vi "Trama_GSA(SubVI).vi"(0 "TRAMA":string) -> (1 "Cluster":T2, 2 "3D fix":string, 3 "Cluster 2":T1)   [LabVIEW 2020]
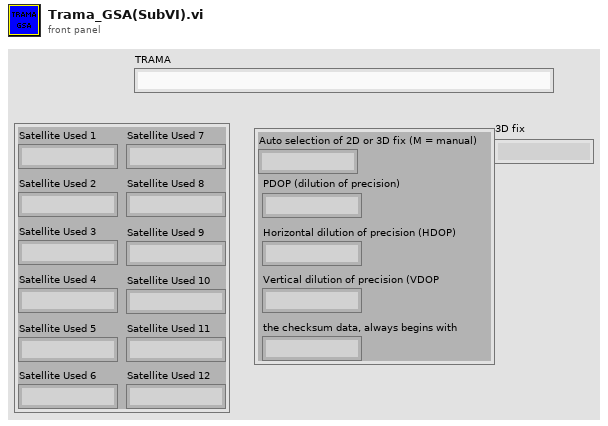
[diagram p1: front panel]
types:
  T1 = cluster{"Satellite Used 1":string, "Satellite Used 2":string, "Satellite Used 3":string, "Satellite Used 4":string, "Satellite Used 5":string, "Satellite Used 6":string, "Satellite Used 7":string, "Satellite Used 8":string, "Satellite Used 9":string, "Satellite Used 10":string, "Satellite Used 11":string, "Satellite Used 12":string}
  T2 = cluster{"Auto selection of 2D or 3D fix (M = manual)":string, "PDOP (dilution of precision)":string, "Horizontal dilution of precision (HDOP)":string, "Vertical dilution of precision (VDOP":string, "the checksum data, always begins with":string}
  T3 = cluster{string, string, string, string, string, string, string, string, string, string, string, string}
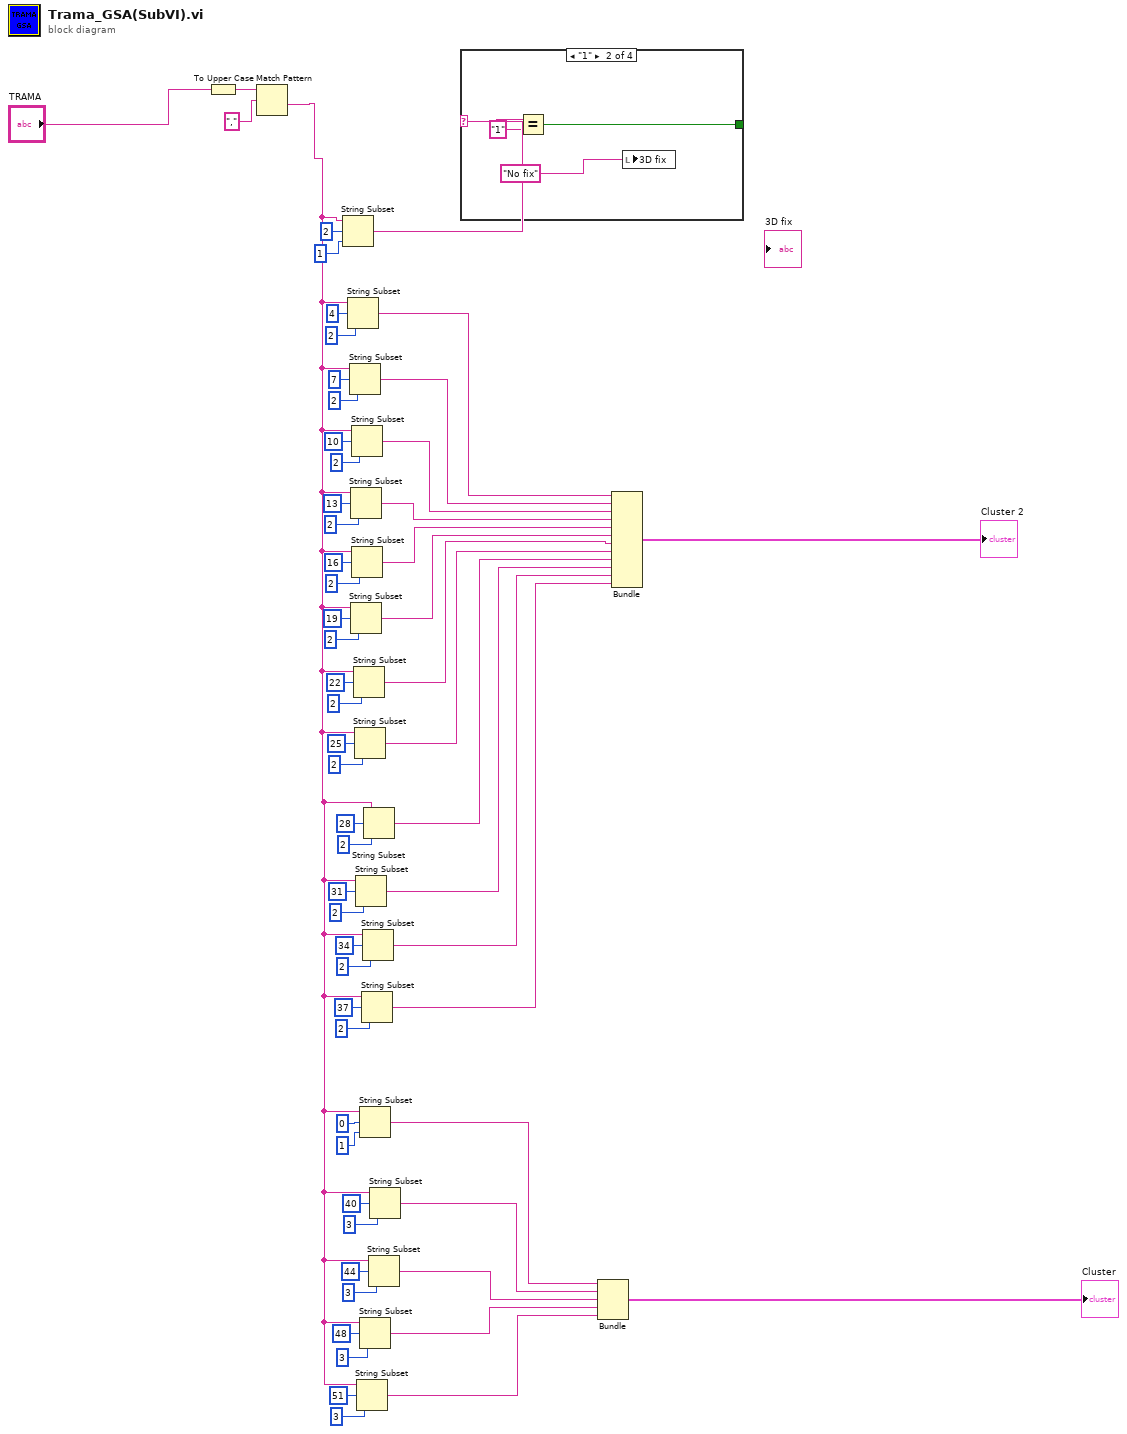
[diagram p0: block diagram]
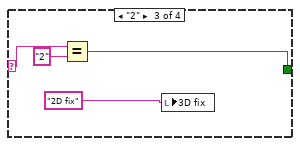
[diagram p3: hidden frame]
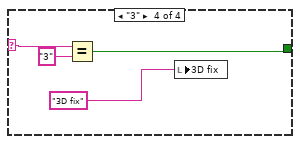
[diagram p4: hidden frame]
diagram:
  n1 = To Upper Case(1:"TRAMA") -> (0:w4:string)
  n2 = Match Pattern(string=w4, regular expression=",") -> (after substring=w58:string)  [unwired: 1 in, 3 out]
  n3 = String Subset(string=w58, offset (0)=2, length (rest)=1 ("length (rest)")) -> (substring=w8:string)
  n4 = String Subset(string=w58, offset (0)=4, length (rest)=2 ("length (rest)")) -> (substring=w39:string)
  n5 = String Subset(string=w58, offset (0)=7, length (rest)=2 ("length (rest)")) -> (substring=w40:string)
  n6 = String Subset(string=w58, offset (0)=13, length (rest)=2 ("length (rest)")) -> (substring=w42:string)
  n7 = String Subset(string=w58, offset (0)=19, length (rest)=2 ("length (rest)")) -> (substring=w44:string)
  n8 = String Subset(string=w58, offset (0)=10, length (rest)=2 ("length (rest)")) -> (substring=w41:string)
  n9 = String Subset(string=w58, offset (0)=16, length (rest)=2 ("length (rest)")) -> (substring=w43:string)
  n10 = String Subset(string=w58, offset (0)=22, length (rest)=2 ("length (rest)")) -> (substring=w45:string)
  n11 = String Subset(string=w58, offset (0)=25, length (rest)=2 ("length (rest)")) -> (substring=w46:string)
  n12 = String Subset(string=w58, offset (0)=31, length (rest)=2 ("length (rest)")) -> (substring=w48:string)
  n13 = String Subset(string=w58, offset (0)=51, length (rest)=3 ("length (rest)")) -> (substring=w55:string)
  n14 = String Subset(string=w58, offset (0)=0, length (rest)=1 ("length (rest)")) -> (substring=w59:string)
  n15 = String Subset(string=w58, offset (0)=48, length (rest)=3 ("length (rest)")) -> (substring=w54:string)
  n16 = String Subset(string=w58, offset (0)=37, length (rest)=2 ("length (rest)")) -> (substring=w50:string)
  n17 = String Subset(string=w58, offset (0)=34, length (rest)=2 ("length (rest)")) -> (substring=w49:string)
  n18 = String Subset(string=w58, offset (0)=28, length (rest)=2 ("length (rest)")) -> (substring=w47:string)
  n19 = String Subset(string=w58, offset (0)=44, length (rest)=3 ("length (rest)")) -> (substring=w53:string)
  n20 = String Subset(string=w58, offset (0)=40, length (rest)=3 ("length (rest)")) -> (substring=w52:string)
  n21 = case shown="\"1\"" w8 {
    selector: w8 -> [_ w64 w66 w71]
    tunnel: [_ w62 w67 w70] -> _
    frame "False", Default {
    }
    frame "1" {
      n22 = Equal?(x=w64, y="1") -> (x = y?=w62:bool)
      n23 = local write "3D fix"("No fix") -> ()
    }
    frame "2" {
      n24 = Equal?(x=w66, y="2") -> (x = y?=w67:bool)
      n25 = local write "3D fix"("2D fix") -> ()
    }
    frame "3" {
      n26 = Equal?(x=w71, y="3") -> (x = y?=w70:bool)
      n27 = local write "3D fix"("3D fix") -> ()
    }
  }
  n28 = Bundle(w59, w52, w53, w54, w55) -> (→"Cluster":cluster{string, string, string, string, string})  [unwired: 1 in]
  n29 = Bundle(w39, w40, w41, w42, w43, w44, w45, w46, w47, w48, w49, w50) -> (→"Cluster 2":T3)  [unwired: 1 in]
